vi "Misc.vi"() -> ()   [LabVIEW 2018]
uses:
  <vilib>/Rock Robotics/Network Tables/NT Read Boolean.vi
  SubSystems/Drive Train/Drive Train Global.vi
  <vilib>/Rock Robotics/Network Tables/NT Write Number.vi
  SubSystems/HAB Climber/HAB Climber Global.vi
  <vilib>/Rock Robotics/Network Tables/NT Write Boolean.vi
  SubSystems/Lift/Lift Global.vi
panel:
  in  "Boolean":bool=TRUE
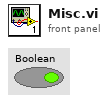
[diagram p1: front panel]
types:
  T1 = typedef "WPI_CompressorDevRef.ctl" = cluster{"DevStatus":errorcluster, "Pneumatics Control Module":u8}
  T2 = cluster{"Rollover":dbl, "Yaw":dbl, "Cont Yaw":dbl}
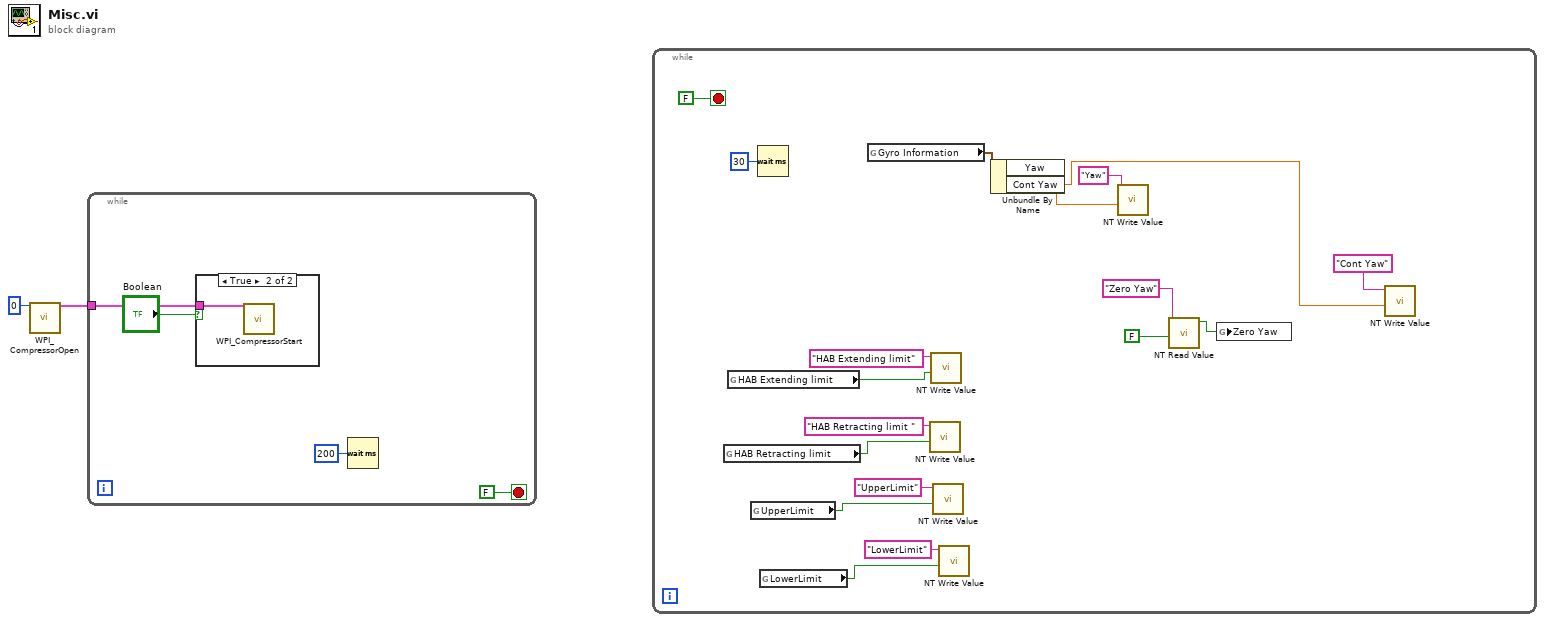
[diagram p0: block diagram]
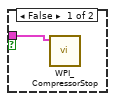
[diagram p2: hidden frame]
diagram:
  n1 = call <vilib>:"WPI_CompressorOpen.vi"("Pneumatics Control Module (0)"=u8 0) -> ("CompressorDevRef"=w1:T1)  [unwired: 13 in, 1 out]
  n2 = while {
    tunnel: w1 -> [w5]
    stop <- FALSE stop-if-true
    n3 = case shown="True" "Boolean" {
      tunnel: w5 -> [w7 w8]
      frame False {
        n4 = call <vilib>:"WPI_CompressorStop.vi"("CompressorDevRef"=w7) -> ()  [unwired: 9 in, 2 out]
      }
      frame True {
        n5 = call <vilib>:"WPI_CompressorStart.vi"("CompressorDevRef"=w8) -> ()  [unwired: 9 in, 2 out]
      }
    }
    n6 = Wait (ms)(milliseconds to wait=u32 200) -> ()  [unwired: 1 out]
  }
  n7 = while {
    stop <- FALSE stop-if-true
    n8 = global read "HAB Climber Global.vi" "HAB Retracting limit"() -> (w12:bool)
    n9 = global read "HAB Climber Global.vi" "HAB Extending limit"() -> (w13:bool)
    n10 = global read "Lift Global.vi" "UpperLimit"() -> (w11:bool)
    n11 = Wait (ms)(milliseconds to wait=u32 30) -> ()  [unwired: 1 out]
    n12 = global read "Lift Global.vi" "LowerLimit"() -> (w10:bool)
    n13 = global read "Drive Train Global.vi" "Gyro Information"() -> (w20:T2)
    n14 = call-poly <vilib>:"NT Write Value.vi"("Boolean"=w12, "Name"="HAB Retracting limit ") -> ()  [unwired: 9 in, 1 out]
    n15 = call-poly <vilib>:"NT Write Value.vi"("Boolean"=w13, "Name"="HAB Extending limit") -> ()  [unwired: 9 in, 1 out]
    n16 = call-poly <vilib>:"NT Write Value.vi"("Boolean"=w11, "Name"="UpperLimit") -> ()  [unwired: 9 in, 1 out]
    n17 = call-poly <vilib>:"NT Write Value.vi"("Boolean"=w10, "Name"="LowerLimit") -> ()  [unwired: 9 in, 1 out]
    n18 = Unbundle By Name(w20) -> ("Yaw"=w19:dbl, "Cont Yaw"=w18:dbl)
    n19 = call-poly <vilib>:"NT Write Value.vi"("Numeric"=w19, "Name"="Yaw") -> ()  [unwired: 9 in, 1 out]
    n20 = call-poly <vilib>:"NT Read Value.vi"("Default Value"=FALSE, "Name"="Zero Yaw") -> ("Boolean"=w21:bool)  [unwired: 8 in, 1 out]
    n21 = global write "Drive Train Global.vi" "Zero Yaw"(w21) -> ()
    n22 = call-poly <vilib>:"NT Write Value.vi"("Numeric"=w18, "Name"="Cont Yaw") -> ()  [unwired: 9 in, 1 out]
  }
